vi "UpdateDIsplayNested.vi"(8 "error in (no error)":errorcluster, 10 "Message":string, 11 "Nested in":refnum<class "Nested.lvclass">) -> (0 "error out":errorcluster, 3 "Nested out":refnum<class "Nested.lvclass">)   [LabVIEW 2020, in "Nested.lvlib" / "Nested.lvclass"]
uses:
  Nested.lvclass
  Nested.lvclass/Nested.ctl
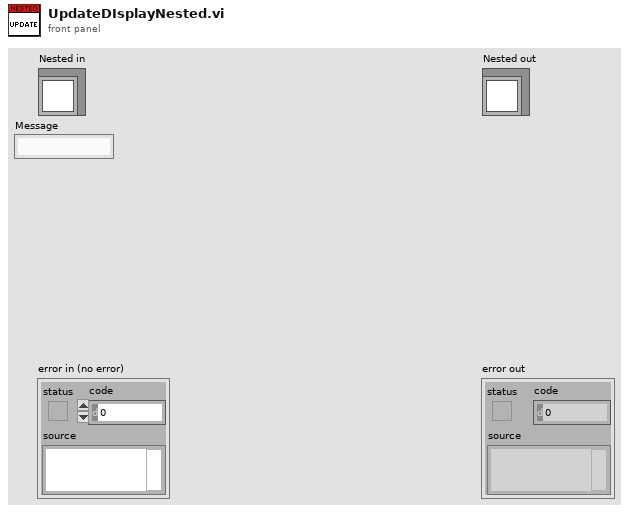
[diagram p1: front panel]
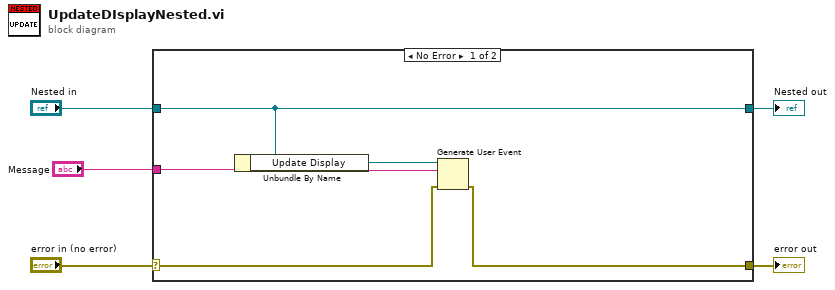
[diagram p0: block diagram]
diagram:
  n1 = case shown="No Error" "error in (no error)" {
    selector: "error in (no error)" -> [w7 w12]
    tunnel: [w6 w12] -> w4
    tunnel: [w10 w11] -> w2
    tunnel: "Nested in" -> [w10 w11]
    tunnel: "Message" -> [w8 _]
    frame No Error {
      n2 = Unbundle By Name(w10) -> ("Update Display"=w9:refnum<user-event>)
      n3 = Generate User Event(user event=w9, event data cluster=w8, error in=w7) -> (error out=w6:errorcluster)  [unwired: 1 in, 1 out]
    }
    frame Error {
    }
  }
  "error out" <- w4
  "Nested out" <- w2
